vi "change CLFN properties.vi"() -> ()   [LabVIEW 2017]
uses:
  <vilib>/Utility/traverseref.llb/TRef TravTarget.ctl
  <userlib>/_OpenG.lib/array/array.llb/Remove Duplicates from 1D Array (String)__ogtk.vi
  <vilib>/Utility/traverseref.llb/VI Scripting - Traverse.lvlib
  <userlib>/_OpenG.lib/array/array.llb/openg_array.lvlib
panel:
  in  "Item(s) to Update":i32[](listbox)
  in  "PGconn/PGresults Type":enum16{"U32", "U64", "Pointer-Size"}(ring)
  out "Functions used":string[](array[string])
  in  "ShowMod":bool=TRUE caption="Open modified diagrams"
  in  "ApplyMod":bool=TRUE caption="Apply modifications"
  in  "Dynamic  Library":bool=TRUE
  in  "Call convention":enum16{"C", "stdcall"}(ring)
  in  "LibPath":string="libpq.*"
  out "Mod":path[](array[path]) caption="Modified VIs"
  in  "AnyThread":bool
  in  "folder":path=path "C:/dev/pq-labview"
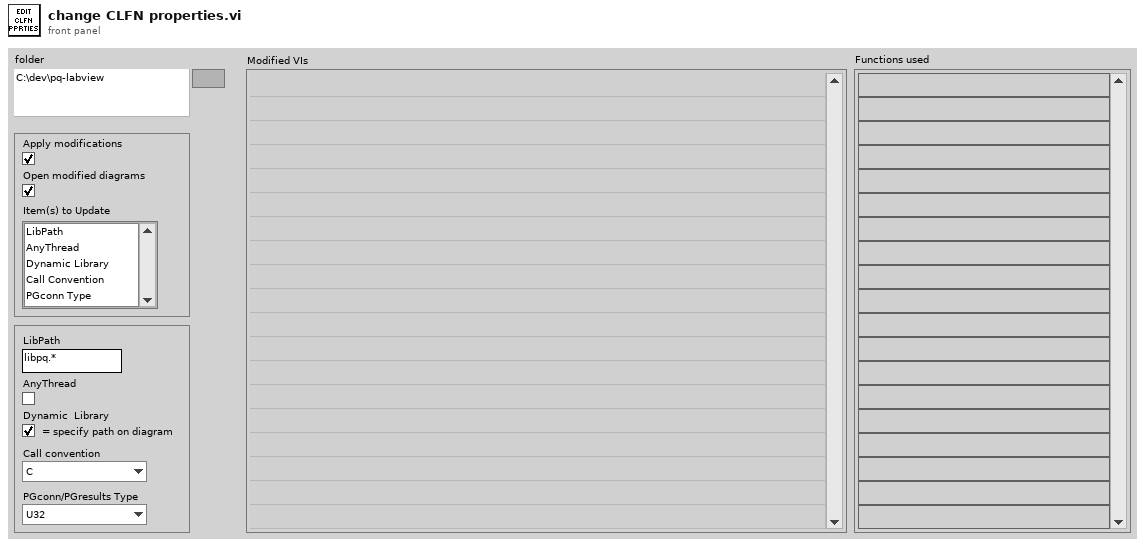
[diagram p1: front panel]
types:
  T1 = cluster{"AnyThread":bool, "LibPath":path, "Call Convention":u32, "Dynamic Library":bool, "PGconn Type":enum16{"I8", "I16", "I32", "I64", "U8", "U16", "U32", "U64", "SGL", "DBL", "PTR INT", "PTR UINT"}}
  T2 = enum16{"I8", "I16", "I32", "I64", "U8", "U16", "U32", "U64", "SGL", "DBL", "PTR INT", "PTR UINT"}
  T3 = typedef "TRef TravTarget.ctl" = enum16{"FP", "BD", "Other"}
  T4 = cluster{"Parameter Name":string, "Num Dimensions":i32, "Parameter Type":enum16{"Numeric", "Array", "String", "Waveform", "Digital Waveform", "Digital Table", "ActiveX", "Any", "Instance Data Pointer", "Void"}, "Numeric Type":enum16{"I8", "I16", "I32", "I64", "U8", "U16", "U32", "U64", "SGL", "DBL", "PTR INT", "PTR UINT"}, "Param Passing":enum16{"By Value", "Pointer To Value"}, "Array Passing":enum16{"Array Data Pointer", "Array Handle", "Array Handle Pointer"}, "String Passing":enum16{"C String Pointer", "Pascal String Pointer", "String Handle", "String Handle Pointer"}, "Adapt Format":enum16{"By Value", "Pointer To Value"}, "ActiveX Types":enum16{"ActiveX Variant Pointer", "IDispatch* Pointer", "IUnknown* Pointer"}, "Const (unused)":bool, "Minimum Size":string}[]
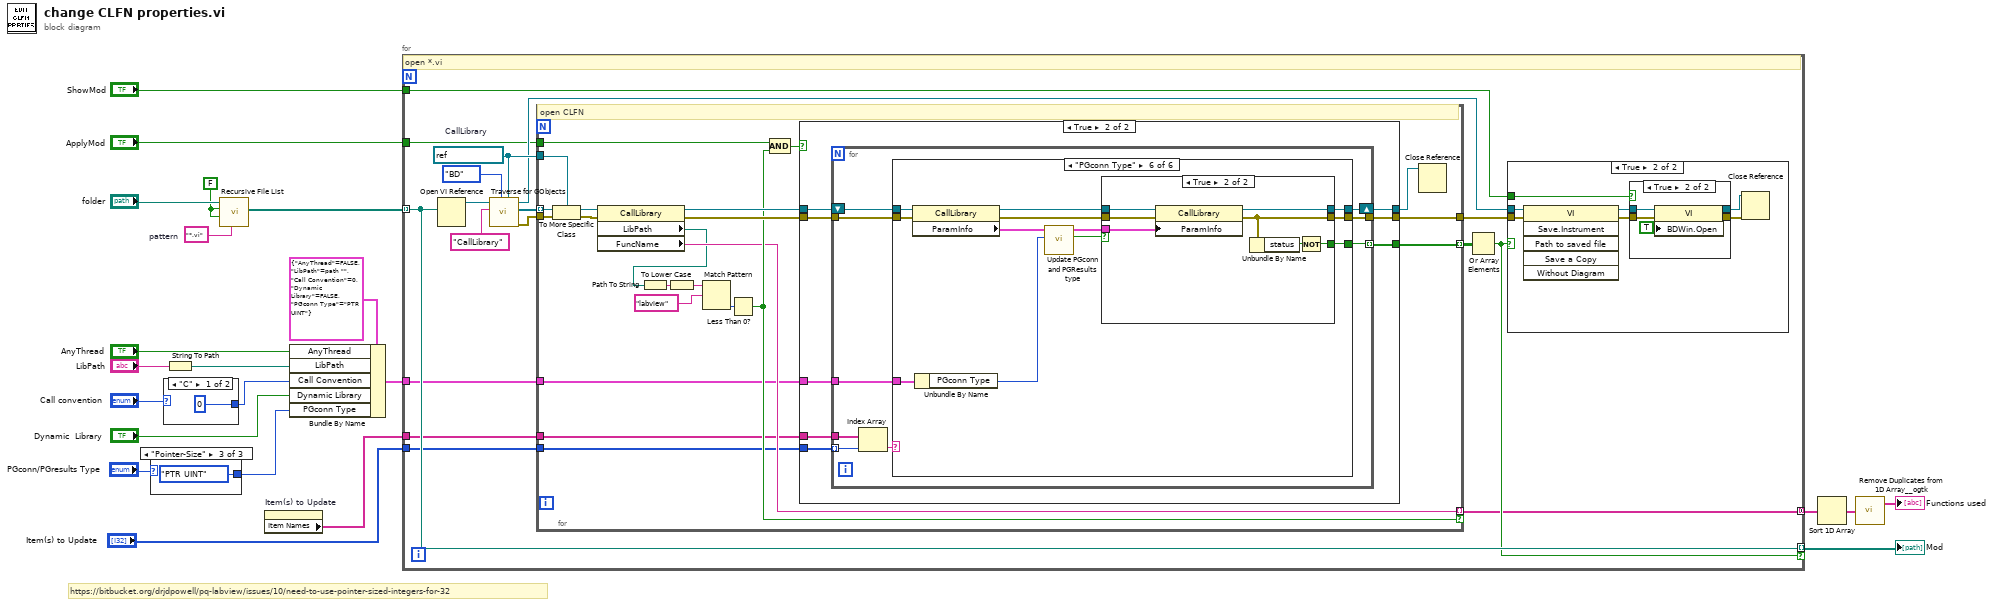
[diagram p0: block diagram]
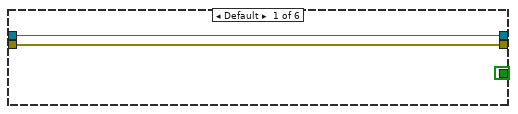
[diagram p3: hidden frame]
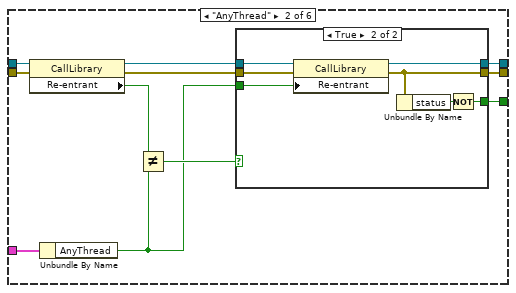
[diagram p4: hidden frame]
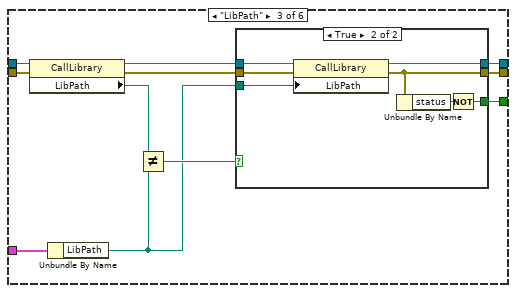
[diagram p6: hidden frame]
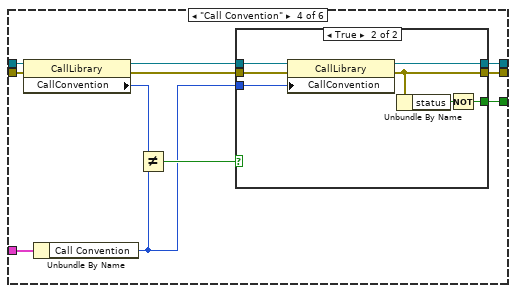
[diagram p8: hidden frame]
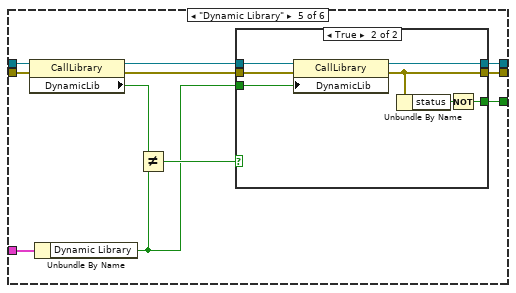
[diagram p10: hidden frame]
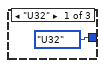
[diagram p15: hidden frame]
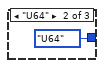
[diagram p16: hidden frame]
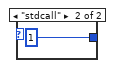
[diagram p17: hidden frame]
diagram:
  w20 = FALSE
  w19 = "*.vi"  # pattern
  # "https://bitbucket.org/drjdpowell/pq-labview/issues/10/need-to-use-pointer-sized-integers-for-32"
  n1 = case shown="\"Pointer-Size\"" "PGconn/PGresults Type" {
    tunnel: [T2."U32" ("Numeric Type") T2."U64" ("Numeric Type") T2."PTR UINT" ("Numeric Type")] -> w4
    frame "U32" {
    }
    frame "U64" {
    }
    frame "Pointer-Size" {
    }
  }
  n2 = case shown="\"C\"" "Call convention" {
    tunnel: [u32 0 ("Calling Convention") u32 1 ("Calling Convention")] -> w6
    frame "C" {
    }
    frame "stdcall" {
    }
  }
  n3 = String To Path(string="LibPath") -> (path=w7:path)
  n4 = call <vilib>:"Recursive File List.vi"("pattern"=w19, "Continue Recursing on Error? (F)"=w20, "Treat LLBs as Folders?"=w20, "Folder Path"="folder") -> ("All Files in Dir"=w18:path[])  [unwired: 3 in, 4 out]
  n5 = property on="Item(s) to Update" class="LstBox (strict)"() -> ("Item Names"=w1:string[])  [unwired: 2 in, 2 out]
  n6 = Bundle By Name(cluster=T1 {"AnyThread"=FALSE, "LibPath"=path "", "Call Convention"=0, "Dynamic Library"=FALSE, "PGconn Type"=enum."PTR UINT"} ("output cluster"), "AnyThread"="AnyThread", "LibPath"=w7, "Call Convention"=w6, "Dynamic Library"="Dynamic  Library", "PGconn Type"=w4) -> (w5:T1)
  n7 = for {
    tunnel: w18 -> [w36] mode=indexing
    tunnel: [w36] -> w22 mode=indexing if=w32
    tunnel: "ApplyMod" -> [w35]
    tunnel: "ShowMod" -> [w34]
    tunnel: [w31] -> w13 mode=concatenating
    tunnel: w5 -> [w30]
    tunnel: "Item(s) to Update" -> [w29]
    tunnel: w1 -> [w28]
    w41 = refnum<vi> refnum  # CallLibrary
    # "open *.vi"
    n8 = Open VI Reference(vi path=w36) -> (vi reference=w44:refnum<vi>)  [unwired: 5 in, 1 out]
    n9 = call <vilib>:"Traverse for GObjects.vi"("Other Refnum"=w41, "Traverse Target"=TRef_TravTarget."BD", "Class Name"="CallLibrary", "VI Refnum"=w44) -> ("error out"=w40:errorcluster, "References"=w37:refnum<vi>[], "dup VI Refnum"=w38:refnum<vi>)  [unwired: 4 in, 1 out]
    n10 = for {
      tunnel: w37 -> [w66] mode=indexing
      tunnel: w41 -> [w65]
      tunnel: w40 -> [w64]
      tunnel: [w63] -> w39
      tunnel: w35 -> [w61]
      tunnel: [w60] -> w33 mode=indexing
      tunnel: [w49] -> w31 mode=indexing if=w50
      tunnel: w30 -> [w47]
      tunnel: w29 -> [w46]
      tunnel: w28 -> [w45]
      # "open CLFN"
      n11 = To More Specific Class(target class=w65, reference=w66, error in=w64) -> (specific class reference=w59:refnum<vi>, error out=w58:errorcluster)
      n12 = property class="CallLibrary"(reference=w59, error in=w58) -> (reference out=w57:refnum<vi>, error out=w56:errorcluster, "LibPath"=w48:path, "FuncName"=w49:string)
      n13 = Path To String(path=w48) -> (string=w55:string)
      n14 = To Lower Case(string=w55) -> (all lower case string=w54:string)
      n15 = Match Pattern(string=w54, regular expression="labview") -> (offset past match=w52:i32)  [unwired: 1 in, 3 out]
      n16 = Less Than 0?(x=w52) -> (x < 0?=w50:bool)
      n17 = Compound Arithmetic op=AND(w61, w50) -> (w51:bool)
      n18 = case shown="True" w51 {
        tunnel: w57 -> [w68 w74]
        tunnel: w56 -> [w67 w73]
        tunnel: [w67 w76] -> w63
        tunnel: [w68 w75] -> w62
        tunnel: [_ w72] -> w60
        tunnel: w47 -> [_ w71]
        tunnel: w46 -> [_ w70]
        tunnel: w45 -> [_ w69]
        frame False {
        }
        frame True {
          n19 = for {
            shift-right: [w84] -> w75
            shift-left: w74 -> [w83]
            tunnel: w73 -> [w82]
            tunnel: [w85] -> w76
            tunnel: [w81] -> w72 mode=indexing
            tunnel: w71 -> [w77]
            tunnel: w70 -> [w79] mode=indexing
            tunnel: w69 -> [w80]
            n20 = Index Array(array=w80, index=w79) -> (element=w78:string)
            n21 = case shown="\"PGconn Type\"" w78 {
              tunnel: [w87 w99 w119 w139 w159 w180] -> w85
              tunnel: [w88 w98 w118 w138 w158 w179] -> w84
              tunnel: w83 -> [w88 w97 w117 w137 w157 w178]
              tunnel: w82 -> [w87 w94 w114 w134 w154 w175]
              tunnel: [FALSE w93 w113 w133 w153 w174] -> w81
              tunnel: w77 -> [_ w92 w111 w131 w151 w171]
              frame Default {
              }
              frame "AnyThread" {
                n22 = property class="CallLibrary"(reference=w97, error in=w94) -> (reference out=w96:refnum<vi>, error out=w95:errorcluster, "Re-entrant"=w91:bool)
                n23 = Unbundle By Name(w92) -> ("AnyThread"=w89:bool)
                n24 = Not Equal?(x=w91, y=w89) -> (x != y?=w90:bool)
                n25 = case shown="True" w90 {
                  tunnel: [w100 w105] -> w99
                  tunnel: [w101 w108] -> w98
                  tunnel: w96 -> [w101 w107]
                  tunnel: w95 -> [w100 w106]
                  tunnel: [_ w103] -> w93
                  tunnel: w89 -> [_ w102]
                  frame False {
                  }
                  frame True {
                    n26 = property class="CallLibrary"(reference=w107, error in=w106, "Re-entrant"=w102) -> (reference out=w108:refnum<vi>, error out=w105:errorcluster)
                    n27 = Unbundle By Name(w105) -> ("status"=w104:bool)
                    n28 = Not(x=w104) -> (.not. x?=w103:bool)
                  }
                }
              }
              frame "LibPath" {
                n29 = property class="CallLibrary"(reference=w117, error in=w114) -> (reference out=w116:refnum<vi>, error out=w115:errorcluster, "LibPath"=w110:path)
                n30 = Unbundle By Name(w111) -> ("LibPath"=w109:path)
                n31 = Not Equal?(x=w110, y=w109) -> (x != y?=w112:bool)
                n32 = case shown="True" w112 {
                  tunnel: [w120 w125] -> w119
                  tunnel: [w121 w128] -> w118
                  tunnel: w116 -> [w121 w127]
                  tunnel: w115 -> [w120 w126]
                  tunnel: [_ w123] -> w113
                  tunnel: w109 -> [_ w122]
                  frame False {
                  }
                  frame True {
                    n33 = property class="CallLibrary"(reference=w127, error in=w126, "LibPath"=w122) -> (reference out=w128:refnum<vi>, error out=w125:errorcluster)
                    n34 = Unbundle By Name(w125) -> ("status"=w124:bool)
                    n35 = Not(x=w124) -> (.not. x?=w123:bool)
                  }
                }
              }
              frame "Call Convention" {
                n36 = property class="CallLibrary"(reference=w137, error in=w134) -> (reference out=w136:refnum<vi>, error out=w135:errorcluster, "CallConvention"=w130:u32)
                n37 = Unbundle By Name(w131) -> ("Call Convention"=w129:u32)
                n38 = Not Equal?(x=w130, y=w129) -> (x != y?=w132:bool)
                n39 = case shown="True" w132 {
                  tunnel: [w140 w145] -> w139
                  tunnel: [w141 w148] -> w138
                  tunnel: w136 -> [w141 w147]
                  tunnel: w135 -> [w140 w146]
                  tunnel: [_ w143] -> w133
                  tunnel: w129 -> [_ w142]
                  frame False {
                  }
                  frame True {
                    n40 = property class="CallLibrary"(reference=w147, error in=w146, "CallConvention"=w142) -> (reference out=w148:refnum<vi>, error out=w145:errorcluster)
                    n41 = Unbundle By Name(w145) -> ("status"=w144:bool)
                    n42 = Not(x=w144) -> (.not. x?=w143:bool)
                  }
                }
              }
              frame "Dynamic Library" {
                n43 = property class="CallLibrary"(reference=w157, error in=w154) -> (reference out=w156:refnum<vi>, error out=w155:errorcluster, "DynamicLib"=w150:bool)
                n44 = Unbundle By Name(w151) -> ("Dynamic Library"=w149:bool)
                n45 = Not Equal?(x=w150, y=w149) -> (x != y?=w152:bool)
                n46 = case shown="True" w152 {
                  tunnel: [w160 w165] -> w159
                  tunnel: [w161 w168] -> w158
                  tunnel: w156 -> [w161 w167]
                  tunnel: w155 -> [w160 w166]
                  tunnel: [_ w163] -> w153
                  tunnel: w149 -> [_ w162]
                  frame False {
                  }
                  frame True {
                    n47 = property class="CallLibrary"(reference=w167, error in=w166, "DynamicLib"=w162) -> (reference out=w168:refnum<vi>, error out=w165:errorcluster)
                    n48 = Unbundle By Name(w165) -> ("status"=w164:bool)
                    n49 = Not(x=w164) -> (.not. x?=w163:bool)
                  }
                }
              }
              frame "PGconn Type" {
                n50 = property class="CallLibrary"(reference=w178, error in=w175) -> (reference out=w177:refnum<vi>, error out=w176:errorcluster, "ParamInfo"=w172:T4)
                n51 = Unbundle By Name(w171) -> ("PGconn Type"=w170:T2)
                n52 = call "Update PGconn and PGResults type.vi"("Numeric Type"=w170, "ParamInfo"=w172) -> ("Change"=w169:bool, "ParamInfo"=w173:T4)  [unwired: 8 in]
                n53 = case shown="True" w169 {
                  tunnel: [w181 w186] -> w180
                  tunnel: [w182 w189] -> w179
                  tunnel: w177 -> [w182 w188]
                  tunnel: w176 -> [w181 w187]
                  tunnel: [_ w184] -> w174
                  tunnel: w173 -> [_ w183]
                  frame False {
                  }
                  frame True {
                    n54 = property class="CallLibrary"(reference=w188, error in=w187, "ParamInfo"=w183) -> (reference out=w189:refnum<vi>, error out=w186:errorcluster)
                    n55 = Unbundle By Name(w186) -> ("status"=w185:bool)
                    n56 = Not(x=w185) -> (.not. x?=w184:bool)
                  }
                }
              }
            }
          }
        }
      }
      n57 = Close Reference(reference=w62) -> ()  [unwired: 1 in, 1 out]
    }
    n58 = Or Array Elements(Boolean array=w33) -> (logical OR=w32:bool)
    n59 = case shown="True" w32 {
      tunnel: w39 -> [_ w196]
      tunnel: w38 -> [_ w195]
      tunnel: w34 -> [_ w190]
      frame False {
      }
      frame True {
        n60 = invoke class="VI" method="Save.Instrument"(reference=w195, error in=w196) -> (reference out=w193:refnum<vi>, error out=w194:errorcluster)  [unwired: 4 in, 4 out]
        n61 = case shown="True" w190 {
          tunnel: w194 -> [w197 w203]
          tunnel: w193 -> [w198 w202]
          tunnel: [w198 w201] -> w192
          tunnel: [w197 w200] -> w191
          frame False {
          }
          frame True {
            n62 = property class="VI"(reference=w202, error in=w203, "BDWin.Open"=TRUE ("Block Diagram Window:Open")) -> (reference out=w201:refnum<vi>, error out=w200:errorcluster)
          }
        }
        n63 = Close Reference(reference=w192, error in (no error)=w191) -> ()  [unwired: 1 out]
      }
    }
  }
  "Mod" <- w22
  n64 = Sort 1D Array(array=w13) -> (sorted array=w12:string[])
  n65 = call-poly <userlib>:"Remove Duplicates from 1D Array__ogtk.vi"("Input Array"=w12) -> ("Output Array"=→"Functions used":string[])  [unwired: 1 out]
